vi "Override Values.vi"(8 "error in (no error)":errorcluster, 10 "Double":dbl, 11 "Array in":dbl[](array[numeric])) -> (0 "error out":errorcluster, 3 "Array out":dbl[](array[numeric]))   [LabVIEW 2014]
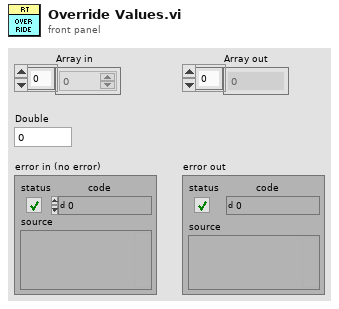
[diagram p1: front panel]
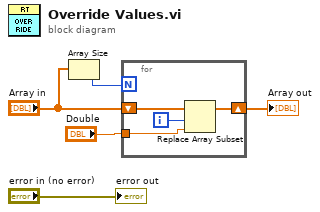
[diagram p0: block diagram]
diagram:
  n1 = Array Size(array="Array in") -> (size(s)=w2:i32)
  n2 = for {
    N: w2 -> [_]
    tunnel: "Double" -> [w9]
    shift-right: [w7] -> w4
    shift-left: "Array in" -> [w6]
    i -> [w8]
    n3 = Replace Array Subset(array=w6, new element=w9, index=w8) -> (w7:dbl[])
  }
  "Array out" <- w4
  "error out" <- "error in (no error)"
